vi "Add Meas Plugin Indicators.vi"(11 "error in (no error)":errorcluster) -> (15 "error out":errorcluster)   [LabVIEW 2021, in "Converter.lvlib"]
uses:
  Converter.lvlib
  Converter Reusables/Converter Reusables.lvlib
  Path Functions/Path Functions.lvlib
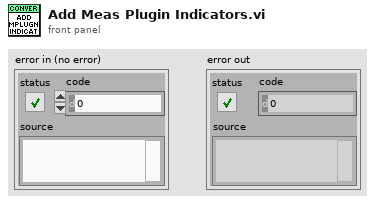
[diagram p1: front panel]
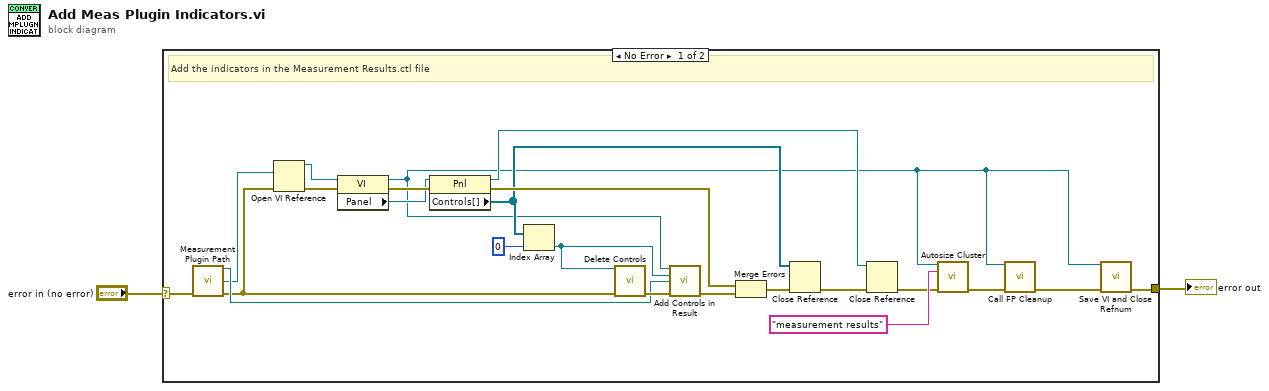
[diagram p0: block diagram]
diagram:
  n1 = case shown="No Error" "error in (no error)" {
    selector: "error in (no error)" -> [w4 w26]
    tunnel: [w18 w26] -> w2
    frame No Error {
      # "Add the indicators in the Measurement Results.ctl file"
      n2 = call "Measurement Plugin Path.vi"("error in (no error)"=w4) -> ("New Code Module"=w6:path, "Result Control"=w5:path, "error out"=w3:errorcluster)  [unwired: 2 in, 10 out]
      n3 = Open VI Reference(vi path=w5, error in (no error)=w3) -> (vi reference=w10:refnum<vi>, error out=w21:errorcluster)  [unwired: 4 in]
      n4 = property class="VI"(reference=w10, error in=w21) -> (reference out=w9:refnum<vi>, error out=w25:errorcluster, "Panel"=w22:refnum<vi>)
      n5 = property class="Pnl"(reference=w22, error in=w25) -> (reference out=w15:refnum<vi>, error out=w14:errorcluster, "Controls[]"=w13:refnum<vi>[])
      n6 = Index Array(array=w13, index=0) -> (element=w8:refnum<vi>)
      n7 = call "Delete Controls.vi"("Control in"=w8, "error in (no error)"=w3) -> ("error out"=w7:errorcluster)  [unwired: 13 in]
      n8 = call "Add Controls in Result.vi"("VI Reference"=w9, "Result Cluster"=w8, "New Code Module"=w6, "error in (no error)"=w7) -> ("error out"=w23:errorcluster)  [unwired: 11 in]
      n9 = Merge Errors(w14, w23) -> (w12:errorcluster)
      n10 = Close Reference(reference=w13, error in (no error)=w12) -> (error out=w11:errorcluster)
      n11 = Close Reference(reference=w15, error in (no error)=w11) -> (error out=w19:errorcluster)
      n12 = call "Autosize Cluster.vi"("VI Refnum"=w9, "name"="measurement results" ("name/order"), "error in (no error)"=w19) -> ("error out"=w17:errorcluster)  [unwired: 12 in]
      n13 = call "Call FP Cleanup.vi"("VI"=w9, "error in (no error)"=w17) -> ("error out"=w16:errorcluster)  [unwired: 13 in]
      n14 = call "Save VI and Close Refnum.vi"("VI Refnum"=w9, "error in"=w16) -> ("error out"=w18:errorcluster)  [unwired: 13 in]
    }
    frame Error {
    }
  }
  "error out" <- w2
